vi "ConvertGoop3ToGoop4_CheckIfNodeIfLinkedToGetAttributeDrains.vi"(1 "FirstGetAttributesDrainsTerminals":refnum<vi>[](array[refnum]), 2 "NodeInfo":T1, 3 "NodesIn":cluster{"NodesIn":T1[]}[](array[cluster])) -> (0 "Boolean":bool)   [LabVIEW 2020]
uses:
  <resource>/Framework/Providers/Open_GDS/ClassProviders/Common/ScriptingFunctions/Scripting_NodeInfo.ctl
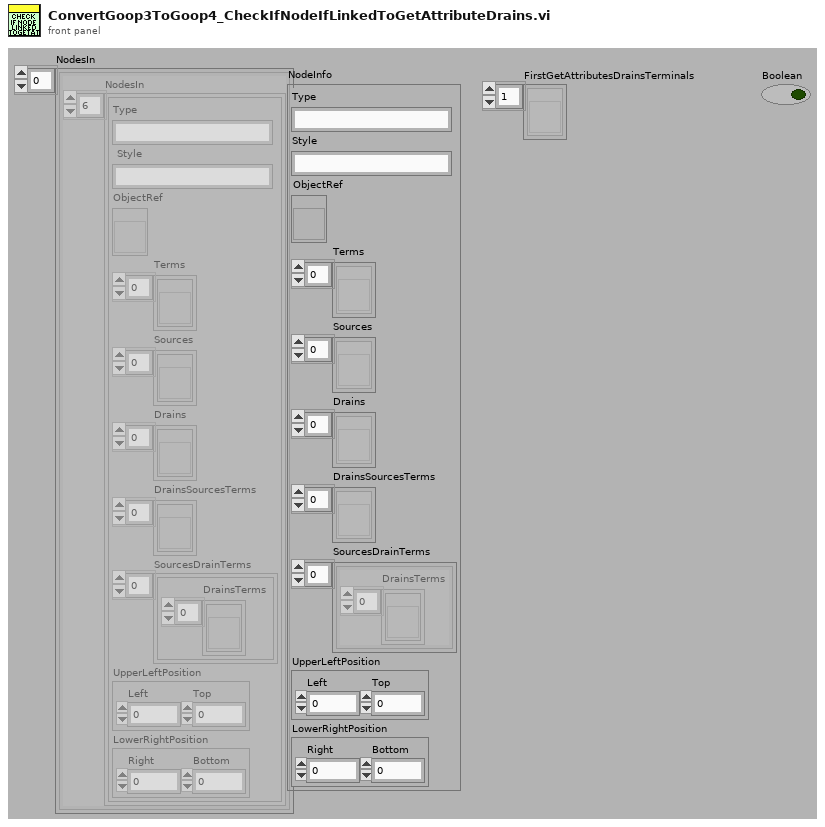
[diagram p1: front panel]
types:
  T1 = typedef "Scripting_NodeInfo.ctl" = cluster{"Type":string, "Style":string, "ObjectRef":refnum<vi>, "Terms":refnum<vi>[], "Sources":refnum<vi>[], "Drains":refnum<vi>[], "DrainsSourcesTerms":refnum<vi>[], "SourcesDrainTerms":cluster{"DrainsTerms":refnum<vi>[]}[], "UpperLeftPosition":cluster{"Left":i32, "Top":i32}, "LowerRightPosition":cluster{"Right":i32, "Bottom":i32}}
  T2 = cluster{"SourcesDrainTerms":cluster{"DrainsTerms":refnum<vi>[]}[]}[]
  T3 = cluster{"SourcesDrainTerms":cluster{"DrainsTerms":refnum<vi>[]}[]}
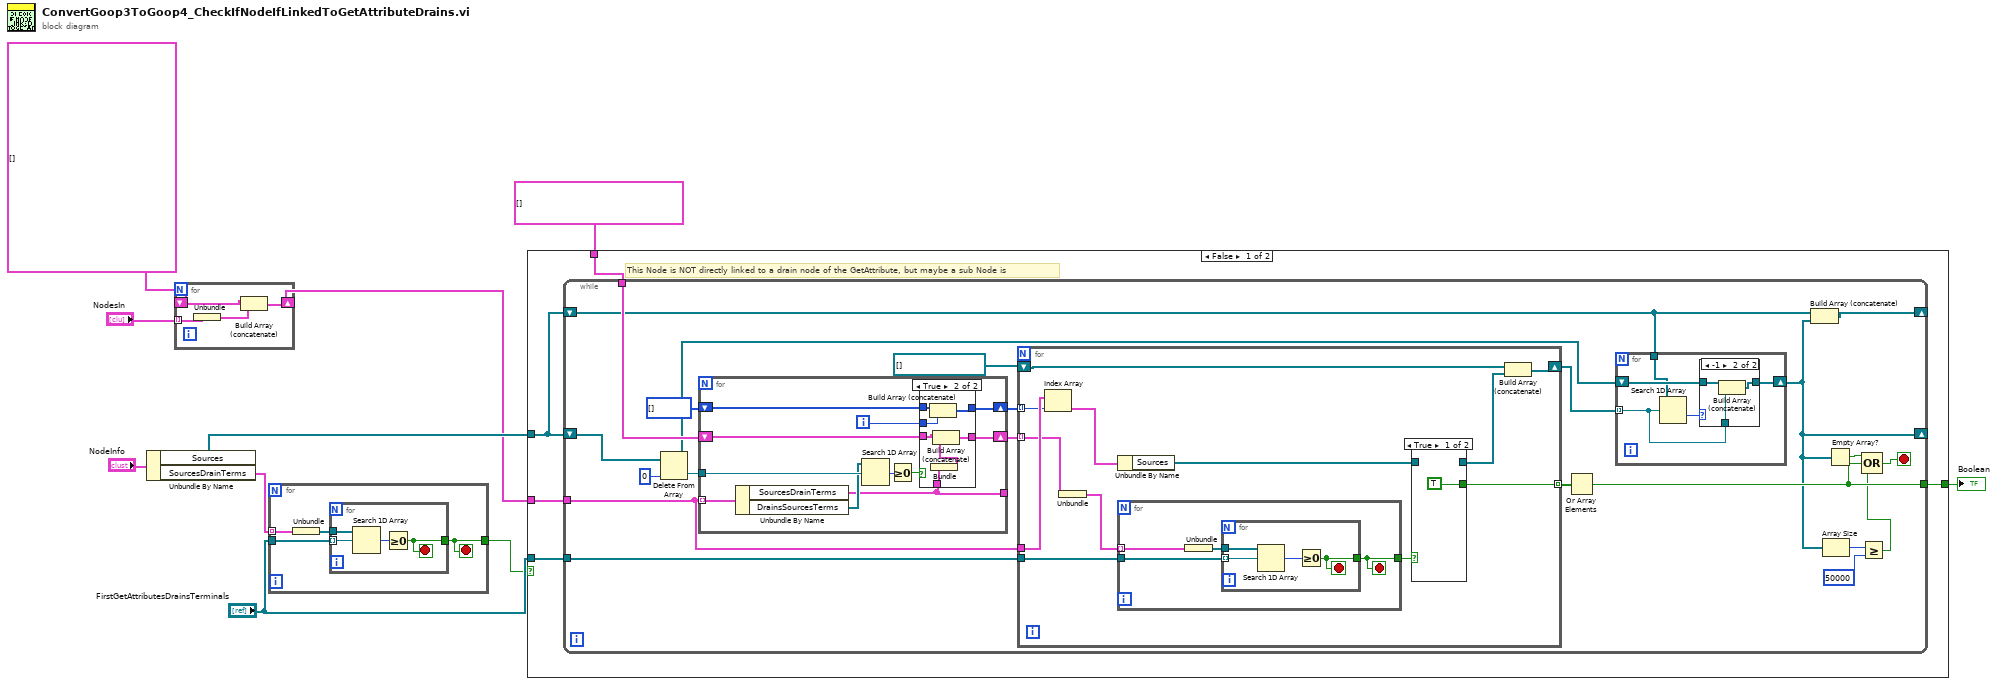
[diagram p0: block diagram]
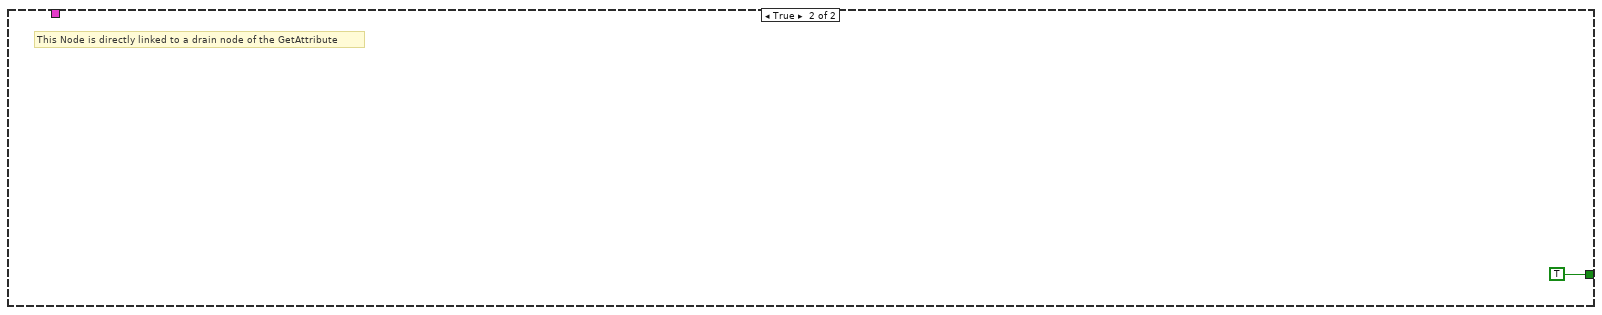
[diagram p5: hidden frame]
diagram:
  n1 = Unbundle By Name("NodeInfo") -> ("Sources"=w6:refnum<vi>[], "SourcesDrainTerms"=w8:cluster{"DrainsTerms":refnum<vi>[]}[])
  n2 = for {
    tunnel: "NodesIn" -> [w14] mode=indexing
    shift-right: [w11] -> w2
    shift-left: T1[] [] -> [w13]
    n3 = Unbundle(w14) -> ("NodesIn"=w12:T1[])
    n4 = Build Array (concatenate)(w13, w12) -> (w11:T1[])
  }
  n5 = for {
    tunnel: w8 -> [w18] mode=indexing
    tunnel: "FirstGetAttributesDrainsTerminals" -> [w16]
    tunnel: [w15] -> w9
    stop <- w15 stop-if-true
    n6 = Unbundle(w18) -> ("DrainsTerms"=w17:refnum<vi>[])
    n7 = for {
      tunnel: w17 -> [w22]
      tunnel: w16 -> [w21] mode=indexing
      tunnel: [w19] -> w15
      stop <- w19 stop-if-true
      n8 = Search 1D Array(1D array=w22, element=w21) -> (index of element=w20:i32)  [unwired: 1 in]
      n9 = Greater Or Equal To 0?(x=w20) -> (x >= 0?=w19:bool)
    }
  }
  n10 = case shown="False" w9 {
    tunnel: w6 -> [w23 _]
    tunnel: [w27 TRUE] -> w7
    tunnel: w2 -> [w26 _]
    tunnel: "FirstGetAttributesDrainsTerminals" -> [w25 _]
    tunnel: T2 [] -> [w24 _]
    frame False {
      # "This Node is NOT directly linked to a drain node of the GetAttribute, but maybe a sub Node is"
      n11 = while {
        tunnel: w26 -> [w47]
        tunnel: [w39] -> w27
        shift-right: [w29] -> _
        shift-left: w23 -> [w37]
        tunnel: w25 -> [w43]
        tunnel: w24 -> [w38]
        shift-right: [w28] -> _
        shift-left: w23 -> [w30]
        stop <- w44 stop-if-true
        n12 = Delete From Array(array=w37, index=0) -> (deleted portion=w48:refnum<vi>, array with subset deleted=w35:refnum<vi>[])  [unwired: 1 in]
        n13 = for {
          tunnel: w47 -> [w91] mode=indexing
          tunnel: w48 -> [w90]
          tunnel: [w83] -> _
          shift-right: [w85] -> w41
          shift-left: i32[] [] -> [w86]
          shift-right: [w81] -> w36
          shift-left: w38 -> [w82]
          i -> [w87]
          n14 = Unbundle By Name(w91) -> ("SourcesDrainTerms"=w83:cluster{"DrainsTerms":refnum<vi>[]}[], "DrainsSourcesTerms"=w88:refnum<vi>[])
          n15 = Search 1D Array(1D array=w88, element=w90) -> (index of element=w89:i32)  [unwired: 1 in]
          n16 = Greater Or Equal To 0?(x=w89) -> (x >= 0?=w84:bool)
          n17 = case shown="True" w84 {
            tunnel: w87 -> [_ w98]
            tunnel: w86 -> [w93 w100]
            tunnel: [w93 w99] -> w85
            tunnel: w83 -> [_ w97]
            tunnel: w82 -> [w92 w96]
            tunnel: [w92 w95] -> w81
            frame False {
            }
            frame True {
              n18 = Build Array (concatenate)(w100, w98) -> (w99:i32[])
              n19 = Bundle("SourcesDrainTerms"=w97) -> (w94:T3)  [unwired: 1 in]
              n20 = Build Array (concatenate)(w96, w94) -> (w95:T2)
            }
          }
        }
        n21 = for {
          tunnel: w47 -> [w70]
          tunnel: [w68] -> w46 mode=indexing
          tunnel: w43 -> [w67]
          tunnel: w41 -> [w66] mode=indexing
          shift-right: [w63] -> w34
          shift-left: refnum<vi>[] [] -> [w65]
          tunnel: w36 -> [w60] mode=indexing
          n22 = Index Array(array=w70, index=w66) -> (element=w69:T1)
          n23 = Unbundle(w60) -> ("SourcesDrainTerms"=w59:cluster{"DrainsTerms":refnum<vi>[]}[])
          n24 = for {
            tunnel: w59 -> [w74] mode=indexing
            tunnel: w67 -> [w72]
            tunnel: [w71] -> w61
            stop <- w71 stop-if-true
            n25 = Unbundle(w74) -> ("DrainsTerms"=w73:refnum<vi>[])
            n26 = for {
              tunnel: w73 -> [w78]
              tunnel: w72 -> [w77] mode=indexing
              tunnel: [w75] -> w71
              stop <- w75 stop-if-true
              n27 = Search 1D Array(1D array=w78, element=w77) -> (index of element=w76:i32)  [unwired: 1 in]
              n28 = Greater Or Equal To 0?(x=w76) -> (x >= 0?=w75:bool)
            }
          }
          n29 = Unbundle By Name(w69) -> ("Sources"=w62:refnum<vi>[])
          n30 = case shown="True" w61 {
            tunnel: [TRUE _] -> w68
            tunnel: [_ w80] -> w64
            tunnel: w62 -> [_ w80]
            frame True {
            }
            frame False {
            }
          }
          n31 = Build Array (concatenate)(w65, w64) -> (w63:refnum<vi>[])
        }
        n32 = Or Array Elements(Boolean array=w46) -> (logical OR=w39:bool)
        n33 = for {
          shift-right: [w53] -> w29
          shift-left: w35 -> [w54]
          tunnel: w34 -> [w51] mode=indexing
          tunnel: w30 -> [w52]
          n34 = Search 1D Array(1D array=w52, element=w51) -> (index of element=w50:i32)  [unwired: 1 in]
          n35 = case shown="-1" w50 {
            tunnel: w54 -> [w55 w58]
            tunnel: [w55 w57] -> w53
            tunnel: w51 -> [_ w56]
            frame 0, Default {
            }
            frame -1 {
              n36 = Build Array (concatenate)(w58, w56) -> (w57:refnum<vi>[])
            }
          }
        }
        n37 = Build Array (concatenate)(w30, w29) -> (w28:refnum<vi>[])
        n38 = Array Size(array=w29) -> (size(s)=w33:i32)
        n39 = Empty Array?(array=w29) -> (empty?=w45:bool)
        n40 = Greater Or Equal?(x=w33, y=50000) -> (x >= y?=w31:bool)
        n41 = Compound Arithmetic op=OR(w45, w39, w31) -> (w44:bool)
      }
    }
    frame True {
      # "This Node is directly linked to a drain node of the GetAttribute"
    }
  }
  "Boolean" <- w7
